vi "2L01-E(X)_s_MIF_n0.vi"(0 "ni":u32[](array[numeric]), 1 "xic":dbl[](array[numeric])) -> (2 "V(X)":dbl, 3 "s":dbl, 4 "E(X)":dbl)   [LabVIEW 2010, in "lv_02.lvlib"]
doc: "Calcul de E(X), V(X) et s à partir d'une distribution xic, ni."
uses:
  lv_02.lvlib
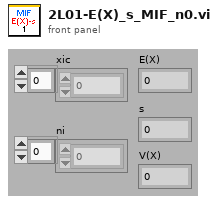
[diagram p1: front panel]
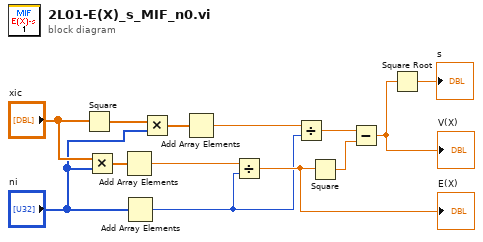
[diagram p0: block diagram]
diagram:
  n1 = Square(x="xic") -> (x^2=w6:dbl[])
  n2 = Multiply(x="xic", y="ni") -> (x*y=w8:dbl[])
  n3 = Add Array Elements(numeric array=w8) -> (sum=w9:dbl)
  n4 = Add Array Elements(numeric array="ni") -> (sum=w1:u32)
  n5 = Multiply(x=w6, y="ni") -> (x*y=w2:dbl[])
  n6 = Add Array Elements(numeric array=w2) -> (sum=w10:dbl)
  n7 = Divide(x=w9, y=w1) -> (x/y=w5:dbl)
  "E(X)" <- w5
  n8 = Divide(x=w10, y=w1) -> (x/y=w11:dbl)
  n9 = Square(x=w5) -> (x^2=w7:dbl)
  n10 = Subtract(x=w11, y=w7) -> (x-y=w3:dbl)
  "V(X)" <- w3
  n11 = Square Root(x=w3) -> (sqrt(x)=→"s":dbl)
